vi "Get_Ch_Strings_from_file.vi"(0 "Filename":path, 9 "Channel names":string[](array[string]), 11 "Start of read offset (chars.: 0)":i32) -> (4 "exists?":bool, 6 "File Channels":string[](array[string]), 15 "Ch Data":string[][](array[string]))   [LabVIEW 2010]
panel:
  in  "stop":bool
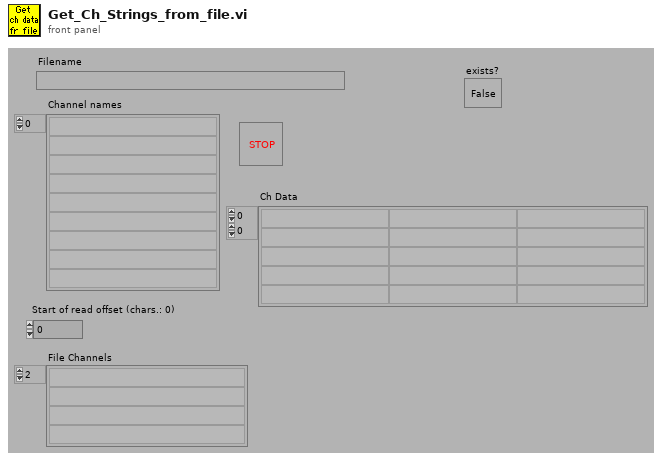
[diagram p1: front panel]
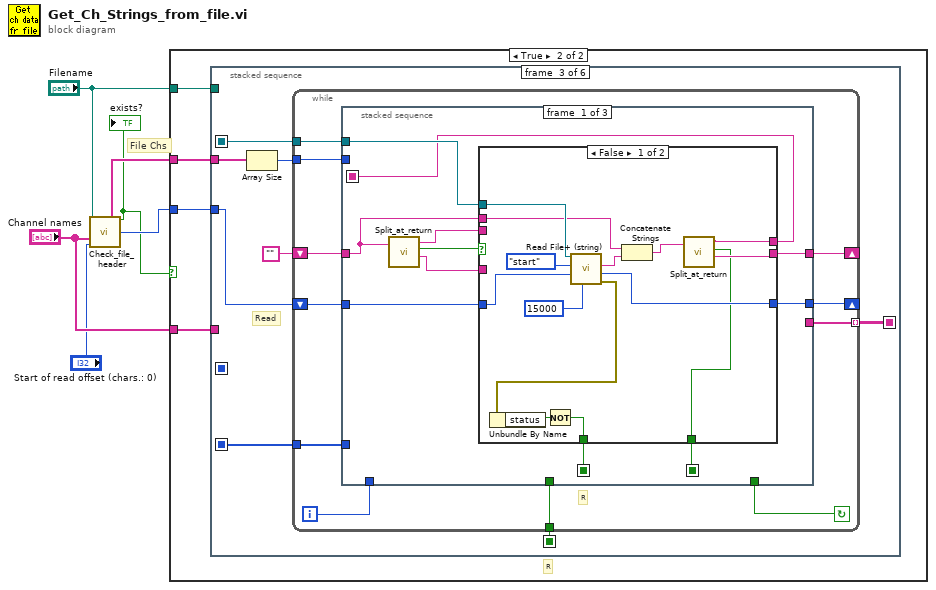
[diagram p0: block diagram]
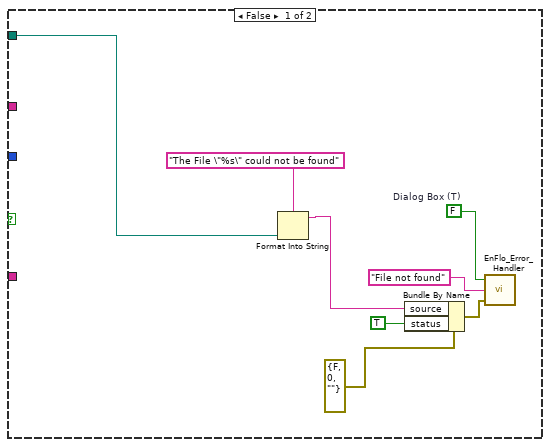
[diagram p2: hidden frame]
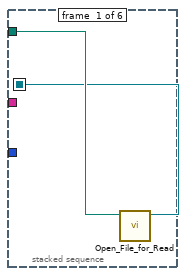
[diagram p3: hidden frame]
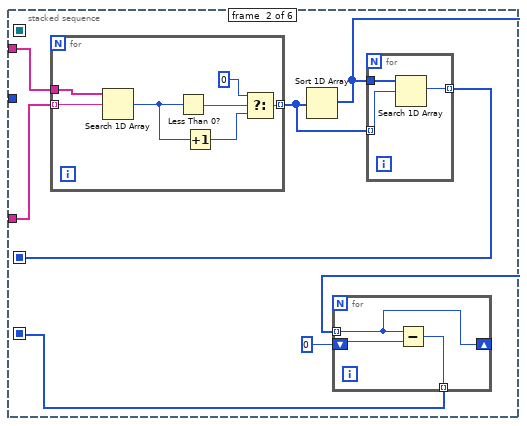
[diagram p4: hidden frame]
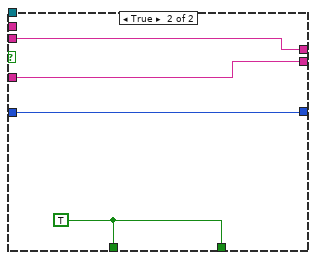
[diagram p5: hidden frame]
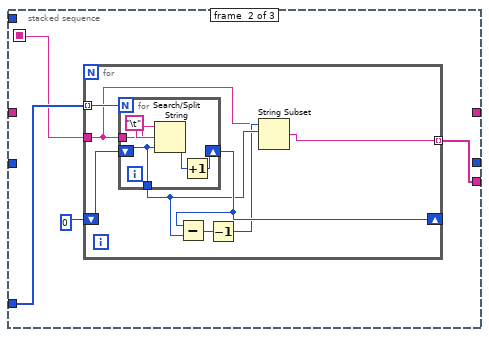
[diagram p6: hidden frame]
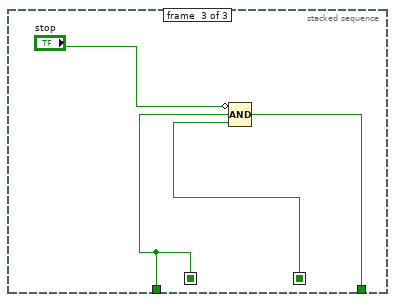
[diagram p7: hidden frame]
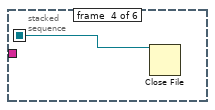
[diagram p8: hidden frame]
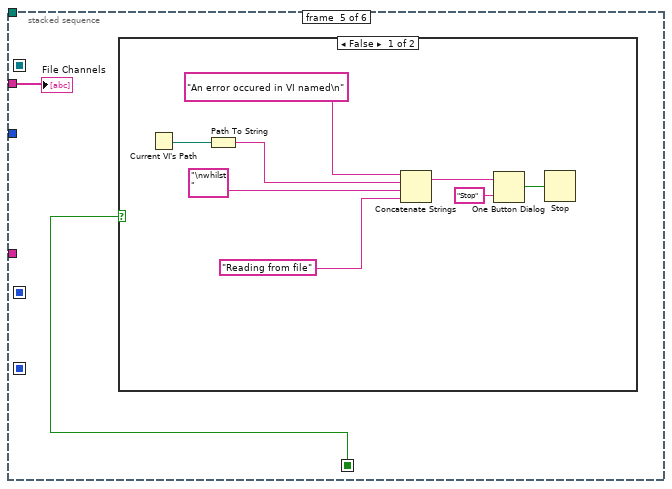
[diagram p9: hidden frame]
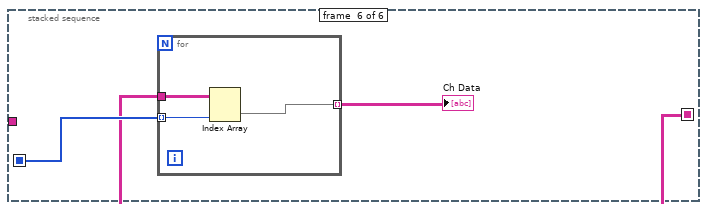
[diagram p11: hidden frame]
diagram:
  # "File Chs"
  n1 = call "Check_file_header.vi"("Filename"="Filename", "Present Channels"="Channel names", "Start of read offset (chars.: 0)"="Start of read offset (chars.: 0)") -> ("File Channels"=w5:string[], "exists?"=w1:bool, "Start of data (bytes)"=w6:i32)  [unwired: 1 in, 9 out]
  "exists?" <- w1
  n2 = case shown="True" w1 {
    tunnel: w6 -> [_ w17]
    tunnel: w5 -> [_ w16]
    tunnel: "Filename" -> [w14 w18]
    tunnel: "Channel names" -> [_ w15]
    frame False {
      w7 = FALSE  # Dialog Box (T)
      n3 = Format Into String(format string="The File \"%s\" could not be found", w14) -> (resulting string=w9:string)  [unwired: 2 in, 1 out]
      n4 = Bundle By Name(cluster=errorcluster {"status"=FALSE, "code"=0, "source"=""} ("error in (no error)"), "source"=w9, "status"=TRUE) -> (w8:errorcluster)
      n5 = call "EnFlo_Error_Handler.vi"("error in (no error)"=w8, "Error Type"="File not found", "Dialog Box (T)"=w7) -> ()  [unwired: 3 out]
    }
    frame True {
      # "R"
      n6 = stacked-sequence {
        seq-local: [w19 _ _ _ _ _] -> [_ _ w47 w110 _ _]
        seq-local: [_ _ w44 _ _ _] -> [_ _ _ _ w112 _]
        seq-local: [_ _ w42 _ _ _] -> [_ _ _ _ _ w122]
        seq-local: [_ w26 _ _ _ _] -> [_ _ w41 _ _ _]
        seq-local: [_ w22 _ _ _ _] -> [_ _ _ _ _ w123]
        tunnel: w18 -> [w20 _ _ _ _ _]
        tunnel: w17 -> [_ _ w46 _ _ _]
        tunnel: w16 -> [_ w25 w43 _ w111 _]
        tunnel: w15 -> [_ w24 _ _ _ _]
        frame #0 {
          n7 = call "Open_File_for_Read.vi"("file path"=w20) -> ("refnum"=w19:refnum<file>)  [unwired: 1 in, 9 out]
        }
        frame #1 {
          n8 = for {
            tunnel: w25 -> [w40]
            tunnel: w24 -> [w39] mode=indexing
            tunnel: [w36] -> w23 mode=indexing
            n9 = Search 1D Array(1D array=w40, element=w39) -> (index of element=w35:i32)  [unwired: 1 out]
            n10 = Less Than 0?(x=w35) -> (x < 0?=w38:bool)
            n11 = Increment(x=w35) -> (x+1=w34:i32)
            n12 = Select(t=0, s=w38, f=w34) -> (s? t:f=w36:i32)
          }
          n13 = Sort 1D Array(array=w23) -> (sorted array=w21:i32[])
          n14 = for {
            shift-right: [w32] -> _
            shift-left: 0 -> [w33]
            tunnel: w21 -> [w32] mode=indexing
            tunnel: [w31] -> w26 mode=indexing
            n15 = Subtract(x=w32, y=w33) -> (x-y=w31:i32)
          }
          n16 = for {
            tunnel: w21 -> [w30]
            tunnel: w23 -> [w29] mode=indexing
            tunnel: [w28] -> w22 mode=indexing
            n17 = Search 1D Array(1D array=w30, element=w29) -> (index of element=w28:i32)  [unwired: 1 out]
          }
        }
        frame #2 {
          # "Read"
          n18 = Array Size(array=w43) -> (size(s)=w45:i32)
          n19 = while {
            tunnel: w41 -> [w49]
            tunnel: [w51] -> w42 mode=indexing
            tunnel: [w52] -> w44
            tunnel: w45 -> [w54]
            tunnel: w47 -> [w56]
            shift-left: w46 -> [w58]
            shift-right: [w57] -> _
            shift-left: "" -> [w59]
            shift-right: [w55] -> _
            i -> [w50]
            stop <- w53 continue-if-true
            # "R"
            n20 = stacked-sequence {
              seq-local: [w64 _ _] -> [_ w89 _]
              seq-local: [w65 _ _] -> [_ _ w106]
              seq-local: [w66 _ _] -> [_ _ w107]
              tunnel: w59 -> [w60 _ _]
              tunnel: w58 -> [w70 _ _]
              tunnel: [w69 _ _] -> w57
              tunnel: w56 -> [w68 _ _]
              tunnel: [w67 _ _] -> w55
              tunnel: w54 -> [_ _ _]
              tunnel: [_ _ w108] -> w53
              tunnel: [_ _ w107] -> w52
              tunnel: [_ w91 _] -> w51
              tunnel: w50 -> [_ _ _]
              tunnel: w49 -> [_ w92 _]
              frame #0 {
                n21 = call "Split_at_return.vi"("String"=w60) -> ("before substring"=w63:string, "Matched?"=w61:bool, "after substring"=w62:string)  [unwired: 1 in, 1 out]
                n22 = case shown="False" w61 {
                  tunnel: w70 -> [w83 w88]
                  tunnel: [w81 w88] -> w69
                  tunnel: w68 -> [w80 _]
                  tunnel: w60 -> [w78 _]
                  tunnel: [w72 w87] -> w67
                  tunnel: w62 -> [_ w87]
                  tunnel: [w75 w86] -> w66
                  tunnel: [w71 w86] -> w65
                  tunnel: [w73 w85] -> w64
                  tunnel: w63 -> [_ w85]
                  frame False {
                    n23 = call <vilib>:"Read File+ (string).vi"("count"=15000, "pos offset (bytes:0)"=w83, "pos mode (rel. to current:2)"=enum16{"start", "end", "current"}."start", "refnum"=w80) -> ("error out"=w77:errorcluster, "mark after read (bytes)"=w81:i32, "string"=w79:string)  [unwired: 1 in, 4 out]
                    n24 = Unbundle By Name(w77) -> ("status"=w76:bool)
                    n25 = Not(x=w76) -> (.not. x?=w75:bool)
                    n26 = Concatenate Strings(w78, w79) -> (w74:string)
                    n27 = call "Split_at_return.vi"("String"=w74) -> ("before substring"=w73:string, "Matched?"=w71:bool, "after substring"=w72:string)  [unwired: 1 in, 1 out]
                  }
                  frame True {
                    w86 = TRUE
                  }
                }
              }
              frame #1 {
                n28 = for {
                  tunnel: w92 -> [w100] mode=indexing
                  tunnel: [w93] -> w91 mode=indexing
                  shift-right: [w98] -> _
                  shift-left: 0 -> [w99]
                  tunnel: w89 -> [w94]
                  n29 = for {
                    N: w100 -> [_]
                    shift-right: [w101] -> w98
                    shift-left: w99 -> [w103]
                    tunnel: w94 -> [w104]
                    tunnel: [w103] -> w97
                    n30 = Search/Split String(string=w104, search string/char (-)="\t", offset (0)=w103) -> (offset of match=w102:i32)  [unwired: 2 out]
                    n31 = Increment(x=w102) -> (x+1=w101:i32)
                  }
                  n32 = Subtract(x=w98, y=w97) -> (x-y=w96:i32)
                  n33 = Decrement(x=w96) -> (x-1=w95:i32)
                  n34 = String Subset(string=w94, offset (0)=w97, length (rest)=w95) -> (substring=w93:string)
                }
              }
              frame #2 {
                n35 = Compound Arithmetic op=AND(invert "stop", w107, w106) -> (w108:bool)
              }
            }
          }
        }
        frame #3 {
          n36 = Close File(refnum=w110) -> ()  [unwired: 1 in, 2 out]
        }
        frame #4 {
          n37 = case shown="False" w112 {
            frame False {
              n38 = Current VI's Path() -> (path=w113:path)
              n39 = Path To String(path=w113) -> (string=w119:string)
              n40 = Concatenate Strings("An error occured in VI named\n", w119, "\nwhilst ", "Reading from file") -> (w117:string)
              n41 = One Button Dialog(message=w117, button name ("OK")="Stop") -> (true=w115:bool)
              n42 = Stop(stop? (T)=w115) -> ()
            }
            frame True {
            }
          }
          "File Channels" <- w111
        }
        frame #5 {
          n43 = for {
            tunnel: w123 -> [w126] mode=indexing
            tunnel: w122 -> [w125]
            tunnel: [w124] -> w121 mode=indexing
            n44 = Index Array(array=w125, index (col)=w126) -> (element=w124:string[])  [unwired: 1 in]
          }
          "Ch Data" <- w121
        }
      }
    }
  }
